vi "Demo Window Movement.vi"() -> ()   [LabVIEW 2021, in "Panel Movement Center Maximize.lvlib"]
doc: "This is a demo showing the various panel movement operations such as maximizing on a specified monitor, or moving the panel to a position centered on the mouse, or centered on the monitor the mouse is on.\n\n-----\nHooovahh\n(Brian Hoover)"
uses:
  <vilib>/Utility/miscctls.llb/LVRectTypeDef.ctl
  Panel Movement Center Maximize.lvlib
panel:
  in  "Enter Pressed":bool
  in  "Tab Control":T1(tab)
  in  "Maximize Mouse":bool
  in  "Window Mode (Center on Monitor)":enum16{"Center on Monitor", "Center on Mouse"}(ring)
  in  "Maximize Monitor":bool
  in  "Method (Maximize on Primary)":T2(ring)
  # "Pressing Enter will also perform the \"Set\" command."
  # "Here we can either move the panel so it centers on the mouse as best it can, but stay in the same monitor.  This should mean  when the mouse is near the edge the window will snap to the sides.\n\nOr it can center on the monitor that the mouse is on."
  # "Here we set the panel to maximize on a specific monitor."
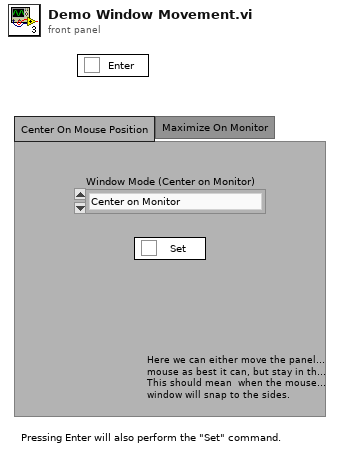
[diagram p1: front panel]
types:
  T1 = enum32{"Center On Mouse Position", "Maximize On Monitor"}
  T2 = enum16{"Maximize on Primary", "Maximize on Secondary", "Maximize on Third", "Maximize on Left", "Maximize on Right", "Maximize Second From Left"}
  T3 = typedef "LVRectTypeDef.ctl" = cluster{"Left":i16, "Top":i16, "Right":i16, "Bottom":i16}
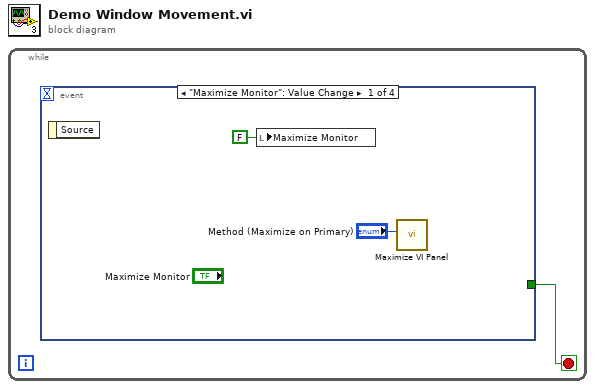
[diagram p0: block diagram]
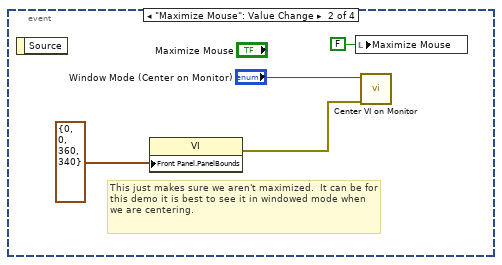
[diagram p2: hidden frame]
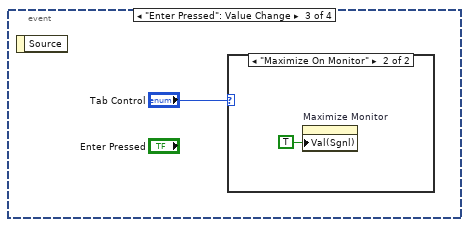
[diagram p3: hidden frame]
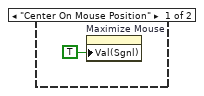
[diagram p4: hidden frame]
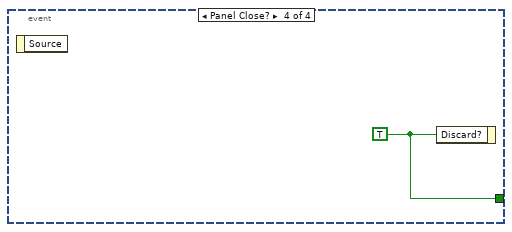
[diagram p5: hidden frame]
diagram:
  n1 = while {
    stop <- w1 stop-if-true
    n2 = event shown="[0] \"Maximize Monitor\": Value Change" {
      selector: _ -> [_ _ _ _]
      dyn-events: _ -> [_ _ _ _]
      timeout: _ -> [_ _ _ _]
      tunnel: [_ _ _ w11] -> w1
      event "Maximize Monitor": Value Change {
        n3 = event-data() -> ()  [unwired: 1 in, 1 out]
        n4 = local write "Maximize Monitor"(FALSE ("Maximize Monitor")) -> ()
        n5 = call "Maximize VI Panel.vi"("Method (Maximize on Primary)"="Method (Maximize on Primary)") -> ()  [unwired: 10 in, 1 out]
      }
      event "Maximize Mouse": Value Change {
        # "This just makes sure we aren't maximized.  It can be for this demo it is best to see it in windowed mode when we are centering."
        n6 = event-data() -> ()  [unwired: 1 in, 1 out]
        n7 = property class="VI"("Front Panel.PanelBounds"=T3 {"Left"=0, "Top"=0, "Right"=360, "Bottom"=340} ("Front Panel Window:Panel Bounds")) -> (error out=w5:errorcluster)  [unwired: 2 in, 1 out]
        n8 = local write "Maximize Mouse"(FALSE ("Maximize Mouse")) -> ()
        n9 = call "Center VI on Monitor.vi"("error in (no error)"=w5, "Window Mode (Center on Monitor)"="Window Mode (Center on Monitor)") -> ()  [unwired: 9 in, 1 out]
      }
      event "Enter Pressed": Value Change {
        n10 = event-data() -> ()  [unwired: 1 in, 1 out]
        n11 = case shown="\"Maximize On Monitor\"" "Tab Control" {
          frame "Center On Mouse Position" {
            n12 = property on="Maximize Mouse" class="Bool (strict)"("Val(Sgnl)"=TRUE ("Value (Signaling)")) -> ()  [unwired: 2 in, 2 out]
          }
          frame "Maximize On Monitor" {
            n13 = property on="Maximize Monitor" class="Bool (strict)"("Val(Sgnl)"=TRUE ("Value (Signaling)")) -> ()  [unwired: 2 in, 2 out]
          }
        }
      }
      event Panel Close? {
        w11 = TRUE ("Discard?")
        n14 = event-data() -> ()  [unwired: 1 in, 1 out]
        n15 = event-data("Discard?"=w11) -> ()  [unwired: 1 in, 1 out]
      }
    }
  }
